vi "Get UI Ref.vi"(8 "error in":errorcluster, 11 "9210 in":refnum<class "9210.lvclass">) -> (0 "error out":errorcluster, 1 "Show SubPanel?":bool, 2 "VI Refnum":refnum<vi>, 3 "9210 out":refnum<class "9210.lvclass">)   [LabVIEW 2019, in "Modules.lvlib" / "9210.lvclass"]
uses:
  9210.lvclass
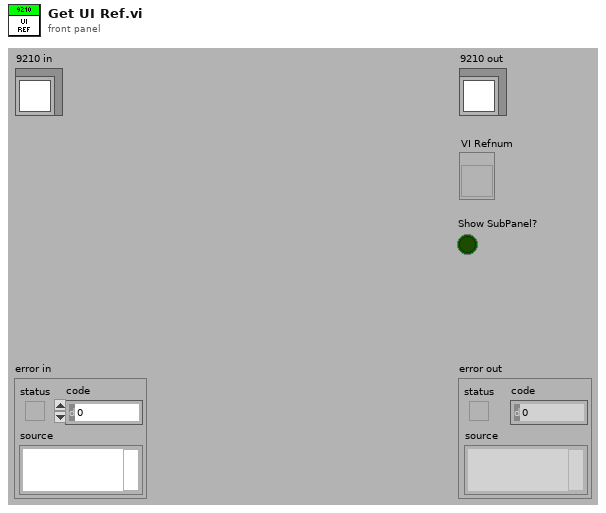
[diagram p1: front panel]
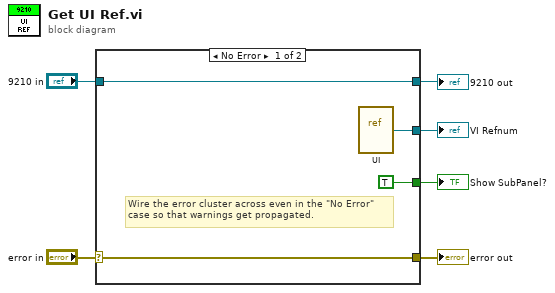
[diagram p0: block diagram]
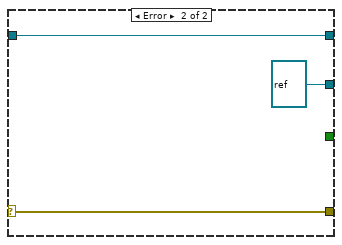
[diagram p2: hidden frame]
diagram:
  n1 = case shown="No Error" "error in" {
    selector: "error in" -> [w9 w13]
    tunnel: [w9 w13] -> w3
    tunnel: [w10 w12] -> w5
    tunnel: "9210 in" -> [w10 w12]
    tunnel: [w8 refnum<vi> refnum] -> w2
    tunnel: [TRUE _] -> w1
    frame No Error {
      # "Wire the error cluster across even in the \"No Error\"\ncase so that warnings get propagated."
      n2 = vi-ref "UI.vi"() -> (w8:refnum<vi>)
    }
    frame Error {
    }
  }
  "error out" <- w3
  "9210 out" <- w5
  "VI Refnum" <- w2
  "Show SubPanel?" <- w1
